vi "NATS CONNECT.vi"(6 "timeout ms (conn default)":i32=-2, 7 "bytes to read (1024)":i32=1024, 8 "error in":errorcluster, 10 "JSON":string="{\"verbose\":false}", 11 "nats connection in":T1={"connection ID"=refnum, "server INFO"="", "timeout ms"=5000, "verbose?"=FALSE, "server headers?"=FALSE, "client headers?"=FALSE}) -> (0 "error out":errorcluster, 1 "CONNECT processed?":bool, 3 "nats connection out":T1={"connection ID"=refnum, "server INFO"="", "timeout ms"=5000, "verbose?"=FALSE, "server headers?"=FALSE, "client headers?"=FALSE})   [LabVIEW 2013, in "NATS Core.lvlib"]
doc: "Sends the CONNECT command to the NATS server. The default message disables verbose mode, a common practice amongst NATS clients written in other languages."
uses:
  NATS Core.lvlib
  Controls/msg type.ctl
  Controls/nats connection.ctl
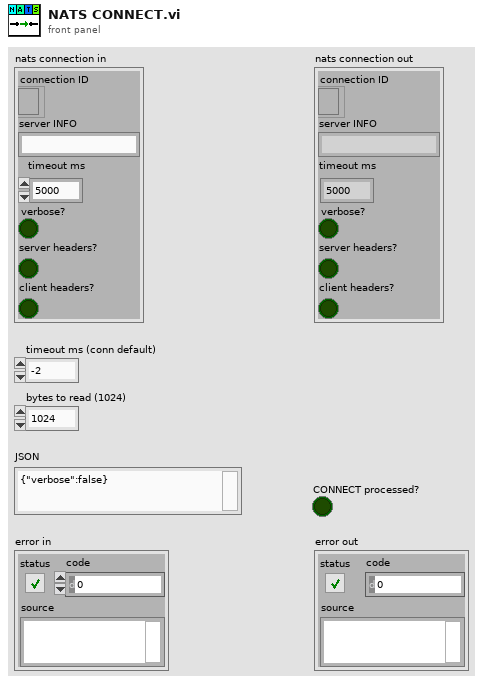
[diagram p1: front panel]
types:
  T1 = typedef "NATS Core.lvlib/nats connection.ctl" = cluster{"connection ID":refnum<k5>, "server INFO":string, "timeout ms":i32, "verbose?":bool, "server headers?":bool, "client headers?":bool}
  T2 = typedef "NATS Core.lvlib/msg type.ctl" = enum16{"Undefined", "MSG", "HMSG", "+OK", "PING", "PONG", "-ERR", "INFO"}
  T3 = typedef "NATS Core.lvlib/nats message.ctl" = cluster{"subject":string, "payload":string, "sub id":string, "reply-to":string, "headers":string, "type":T2, "received":timestamp}
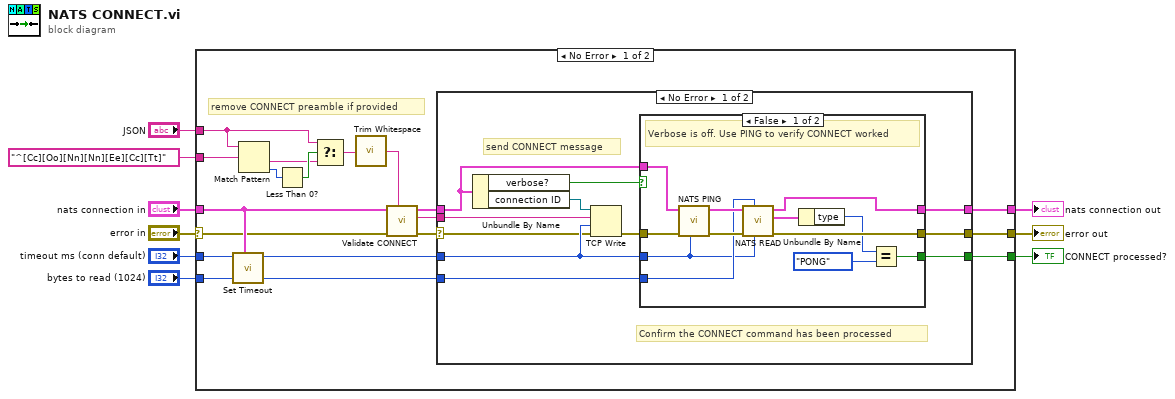
[diagram p0: block diagram]
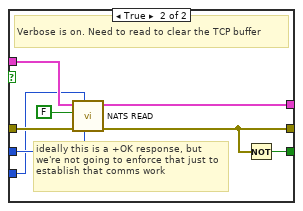
[diagram p2: hidden frame]
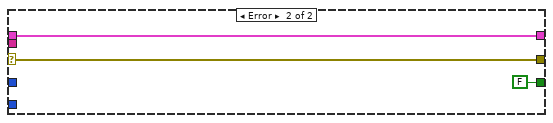
[diagram p3: hidden frame]
diagram:
  n1 = case shown="No Error" "error in" {
    selector: "error in" -> [w19 w63]
    tunnel: "bytes to read (1024)" -> [w26 _]
    tunnel: "timeout ms (conn default)" -> [w22 _]
    tunnel: [w27 w63] -> w7
    tunnel: [w23 w62] -> w5
    tunnel: "JSON" -> [w15 _]
    tunnel: [w24 _] -> w3
    tunnel: "nats connection in" -> [w20 w62]
    tunnel: "^[Cc][Oo][Nn][Nn][Ee][Cc][Tt]" ("string") -> [w10 _]
    frame No Error {
      # "remove CONNECT preamble if provided"
      n2 = call "Set Timeout.vi"("nats connection in"=w20, "timeout ms in"=w22) -> ("timeout ms out"=w21:i32)  [unwired: 9 in]
      n3 = Match Pattern(string=w15, regular expression=w10) -> (after substring=w12:string, offset past match=w17:i32)  [unwired: 1 in, 2 out]
      n4 = Less Than 0?(x=w17) -> (x < 0?=w16:bool)
      n5 = Select(t=w15, s=w16, f=w12) -> (s? t:f=w13:string)
      n6 = call <vilib>:"Trim Whitespace.vi"("string"=w13) -> ("trimmed string"=w11:string)  [unwired: 1 in]
      n7 = call "Validate CONNECT.vi"("JSON"=w11, "error in"=w19, "nats connection in"=w20) -> ("error out"=w18:errorcluster, "CONNECT msg"=w14:string, "nats connection out"=w25:T1)  [unwired: 6 in]
      n8 = case shown="No Error" w18 {
        selector: w18 -> [w28 w60]
        tunnel: [w38 w60] -> w27
        tunnel: w26 -> [w37 _]
        tunnel: w25 -> [w36 w61]
        tunnel: [w35 FALSE] -> w24
        tunnel: [w34 w61] -> w23
        tunnel: w21 -> [w33 _]
        tunnel: w14 -> [w32 _]
        frame No Error {
          # "send CONNECT message"
          # "Confirm the CONNECT command has been processed"
          n9 = Unbundle By Name(w36) -> ("verbose?"=w29:bool, "connection ID"=w30:refnum<k5>)
          n10 = TCP Write(connection ID=w30, data in=w32, error in (no error)=w28, 9:w33) -> (error out=w31:errorcluster)  [unwired: 2 out]
          n11 = case shown="False" w29 {
            tunnel: w31 -> [w48 w56]
            tunnel: [w43 w54] -> w38
            tunnel: w37 -> [w40 w51]
            tunnel: w33 -> [w39 w52]
            tunnel: w36 -> [w45 w57]
            tunnel: [w49 w58] -> w35
            tunnel: [w44 w55] -> w34
            frame False {
              # "Verbose is off. Use PING to verify CONNECT worked"
              n12 = call "NATS PING.vi"("timeout ms (conn default)"=w39, "error in"=w48, "nats connection in"=w45) -> ("error out"=w46:errorcluster, "dup nats connection"=w47:T1)  [unwired: 7 in]
              n13 = call "NATS READ.vi"("timeout ms (conn default)"=w39, "bytes to read (1024)"=w40, "error in"=w46, "nats connection in"=w47) -> ("error out"=w43:errorcluster, "nats message"=w42:T3, "nats connection out"=w44:T1)  [unwired: 4 in, 1 out]
              n14 = Unbundle By Name(w42) -> ("type"=w41:T2)
              n15 = Equal?(x=w41, y=msg_type."PONG") -> (x = y?=w49:bool)
            }
            frame True {
              # "ideally this is a +OK response, but we're not going to enforce that just to establish that comms work"
              # "Verbose is on. Need to read to clear the TCP buffer"
              n16 = call "NATS READ.vi"("timeout ms (conn default)"=w52, "bytes to read (1024)"=w51, "error in"=w56, "suppress timeout error? (T)"=FALSE, "nats connection in"=w57) -> ("error out"=w54:errorcluster, "nats connection out"=w55:T1)  [unwired: 3 in, 2 out]
              n17 = Not(x=w54) -> (.not. x?=w58:bool)
            }
          }
        }
        frame Error {
        }
      }
    }
    frame Error {
    }
  }
  "error out" <- w7
  "nats connection out" <- w5
  "CONNECT processed?" <- w3
